vi "kim18_solution.vi"(6 "6DOF Calibration":T2, 8 "Hemisphere":i32=1, 11 "Coupling magnitude":dbl[][](array[numeric])) -> (3 "Pose transform":T1)   [LabVIEW 2024]
uses:
  <vilib>/Analysis/NI_AALBase.lvlib
  <vilib>/Analysis/NI_AALPro.lvlib
  <vilib>/Analysis/baseanly.llb/Real Inverse Matrix.vi
  <vilib>/Analysis/baseanly.llb/Real A x B.vi
  <vilib>/Analysis/Matrix/Datatypes/RealMatrix.ctl
  <vilib>/Analysis/Matrix/NI_Matrix.lvlib
  <vilib>/Analysis/7linalg.llb/Real SVD Decomposition.vi
  <vilib>/Analysis/Matrix/Numeric/Conversions/Array To Matrix - RA.vi
  6dof_calibration.ctl
panel:
  # "Hemisphere of the source that sensor is located in.\n1, 2, 3 = +X, +Y, +Z hemispheres\n-1, -2, -3 are the negative hemispheres\nThis is the same notation as in the Matlab code"
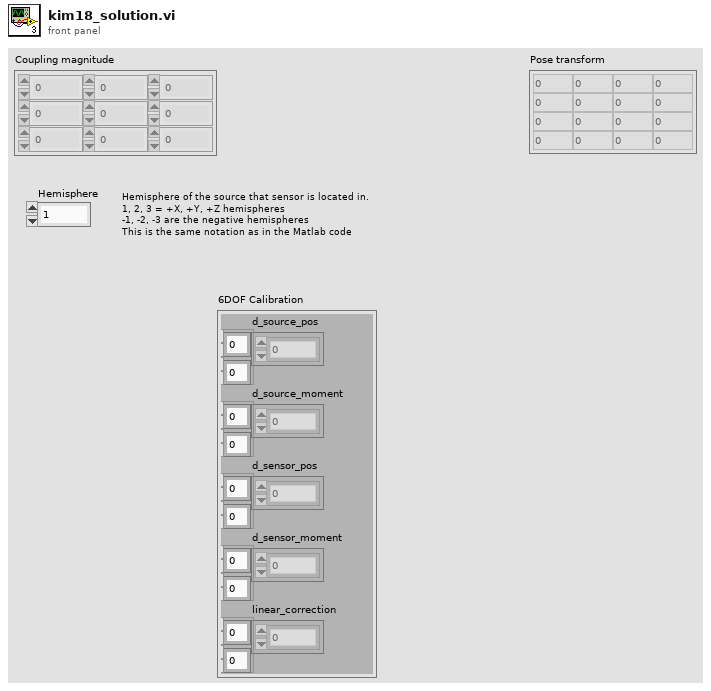
[diagram p1: front panel]
types:
  T1 = typedef "NI_Matrix.lvlib/RealMatrix.ctl" = dbl[][]
  T2 = typedef "6dof_calibration.ctl" = cluster{"d_source_pos":dbl[][], "d_source_moment":dbl[][], "d_sensor_pos":dbl[][], "d_sensor_moment":dbl[][], "linear_correction":dbl[][]}
  T3 = typedef "kim18_calibration.ctl" = cluster{"coupling_gains":T1, "N_":T1, "M_":T1, "mu_":dbl}
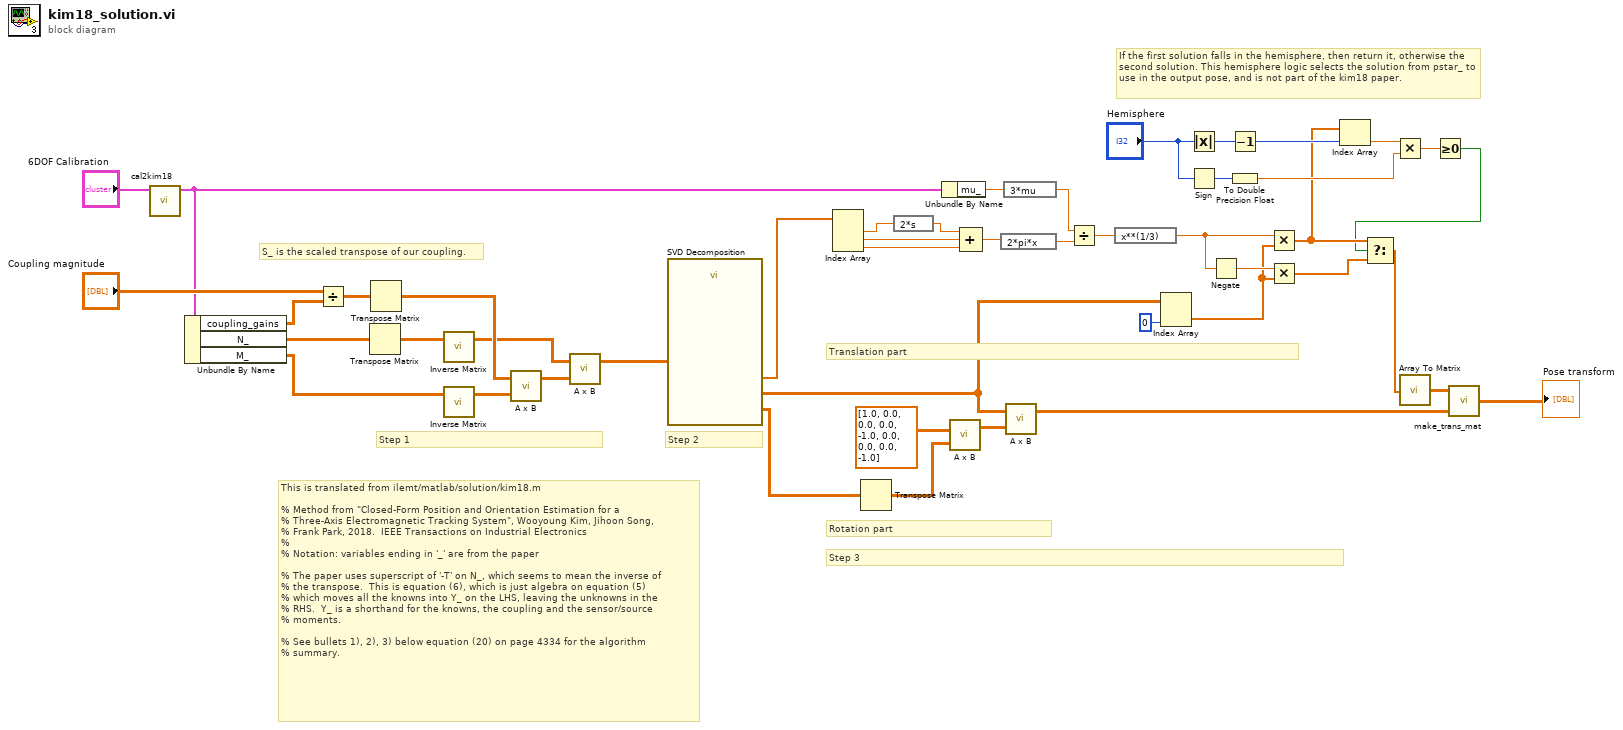
[diagram p0: block diagram]
diagram:
  # "S_ is the scaled transpose of our coupling."
  # "Step 3"
  # "Step 2"
  # "Step 1"
  # "This is translated from ilemt/matlab/solution/kim18.m\n\n% Method from \"Closed-Form Position and Orientation Estimation for a\n% Three-Axis Electromagnetic Tracking System\", Wooyoung Kim, Jihoon Song,\n% Frank Park, 2018.  IEEE Transactions on Industrial Electronics\n%\n% Notation: variables ending in '_' are from the paper\n\n% The paper uses superscript of '-T' on N_, which seems to mean the inverse of\n% the transpose.  This is equation (6), which is just algebra on equation (5)\n% which moves all the knowns into Y_ on the LHS, leaving the unknowns in the\n% RHS.  Y_ is a shorthand for the knowns, the coupling and the sensor/source\n% moments.\n\n% See bullets 1), 2), 3) below equation (20) on page 4334 for the algorithm\n% summary."
  # "Rotation part"
  # "Translation part"
  # "If the first solution falls in the hemisphere, then return it, otherwise the second solution. This hemisphere logic selects the solution from pstar_ to use in the output pose, and is not part of the kim18 paper."
  n1 = call "cal2kim18.vi"("6DOF Calibration"="6DOF Calibration") -> ("Kim18 calibration"=w27:T3)  [unwired: 10 in]
  n2 = Unbundle By Name(w27) -> ("coupling_gains"=w44:T1, "N_"=w42:T1, "M_"=w40:T1)
  n3 = Divide(x="Coupling magnitude", y=w44) -> (x/y=w43:T1)
  n4 = Transpose Matrix(1:w42) -> (0:w41:T1)
  n5 = Transpose Matrix(1:w43) -> (0:w39:T1)
  n6 = call-poly <vilib>:"Inverse Matrix.vi"("Input Matrix"=w41) -> ("Inverse Matrix"=w36:T1)  [unwired: 1 in, 1 out]
  n7 = call-poly <vilib>:"Inverse Matrix.vi"("Input Matrix"=w40) -> ("Inverse Matrix"=w38:T1)  [unwired: 1 in, 1 out]
  n8 = call-poly <vilib>:"A x B.vi"("B"=w38, "A"=w39) -> ("A x B"=w37:T1)  [unwired: 1 out]
  n9 = call-poly <vilib>:"A x B.vi"("B"=w37, "A"=w36) -> ("A x B"=w35:T1)  [unwired: 1 out]
  n10 = call-poly <vilib>:"SVD Decomposition.vi"("A"=w35) -> ("Matrix V"=w19:T1, "Matrix U"=w33:T1, "Vector S"=w30:dbl[])  [unwired: 6 in, 2 out]
  n11 = Index Array(array=w30) -> (element #1=w29:dbl, element #2=w22:dbl, element #3=w21:dbl)  [unwired: 3 in]
  n12 = Transpose Matrix(1:w33) -> (0:w32:T1)
  n13 = expression code="2*s"(w29) -> (w23:dbl)
  n14 = Unbundle By Name(w27) -> ("mu_"=w26:dbl)
  n15 = call-poly <vilib>:"A x B.vi"("B"=w32, "A"=T1 [[1.0, 0.0, 0.0], [0.0, -1.0, 0.0], [0.0, 0.0, -1.0]] ("A x B")) -> ("A x B"=w31:T1)  [unwired: 1 out]
  n16 = Compound Arithmetic op=ADD(w23, w22, w21) -> (w24:dbl)
  n17 = expression code="2*pi*x"(w24) -> (w28:dbl)
  n18 = expression code="3*mu"(w26) -> (w25:dbl)
  n19 = call-poly <vilib>:"A x B.vi"("B"=w31, "A"=w19) -> ("A x B"=w14:T1)  [unwired: 1 out]
  n20 = Divide(x=w25, y=w28) -> (x/y=w20:dbl)
  n21 = expression code="x**(1/3)"(w20) -> (w17:dbl)
  n22 = Index Array(array=w19, index (col)=0 ("disabled index (col)")) -> (element=w15:dbl[])  [unwired: 1 in]
  n23 = Absolute Value(x="Hemisphere") -> (abs(x)=w12:i32)
  n24 = Sign(1:"Hemisphere") -> (0:w11:i32)
  n25 = Negate(x=w17) -> (-x=w16:dbl)
  n26 = Decrement(x=w12) -> (x-1=w10:i32)
  n27 = To Double Precision Float(number=w11) -> (double precision float=w8:dbl)
  n28 = Multiply(x=w17, y=w15) -> (x*y=w5:dbl[])
  n29 = Multiply(x=w16, y=w15) -> (x*y=w6:dbl[])
  n30 = Index Array(array=w5, index=w10) -> (element=w9:dbl)
  n31 = Multiply(x=w9, y=w8) -> (x*y=w7:dbl)
  n32 = Greater Or Equal To 0?(x=w7) -> (x >= 0?=w4:bool)
  n33 = Select(t=w5, s=w4, f=w6) -> (s? t:f=w3:dbl[])
  n34 = call-poly <vilib>:"Array To Matrix.vi"("Real 1D Array"=w3) -> ("Real Matrix (Column Vector)"=w2:T1)
  n35 = call "make_trans_mat.vi"("Rotation"=w14, "Translation"=w2) -> ("Transform"=→"Pose transform":T1)  [unwired: 3 in]
